vi "Write to file.vi"(10 "file path (use dialog)":path, 11 "String":string) -> ()   [LabVIEW 2019]
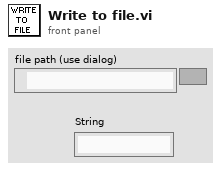
[diagram p1: front panel]
types:
  T1 = enum16{"open", "replace", "create", "open or create", "replace or create", "replace or create with confirmation"}
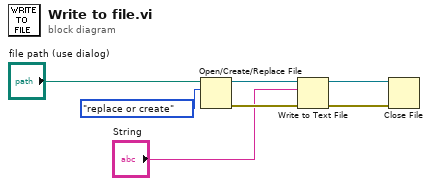
[diagram p0: block diagram]
diagram:
  n1 = Open/Create/Replace File(file path (use dialog)="file path (use dialog)", operation (0:open)=T1."replace or create") -> (refnum out=w3:refnum<file>, error out=w2:errorcluster)  [unwired: 4 in, 1 out]
  n2 = Write to Text File(file (use dialog)=w3, text="String", error in=w2) -> (refnum out=w5:refnum<file>, error out=w4:errorcluster)  [unwired: 1 in, 1 out]
  n3 = Close File(refnum=w5, error in=w4) -> ()  [unwired: 2 out]
